vi "SetupFifo.vi"(8 "Force Num Array":i32, 9 "MaxNumFileWrite":i32=255, 10 "Fifo Time Out":i32=500, 11 "Fifo Size":u32=8192) -> (3 "Data Logging Param":T1)   [LabVIEW 2010, in "kevLib2010.lvlib"]
uses:
  kevLib2010.lvlib
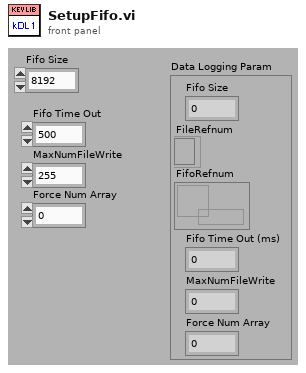
[diagram p1: front panel]
types:
  T1 = cluster{"Fifo Size":u32, "FileRefnum":refnum<file>, "FifoRefnum":refnum<k33>, "Fifo Time Out (ms)":i32, "MaxNumFileWrite":i32, "Force Num Array":i32}
  T2 = enum16{"open", "replace", "create", "open or create", "replace or create", "replace or create with confirmation"}
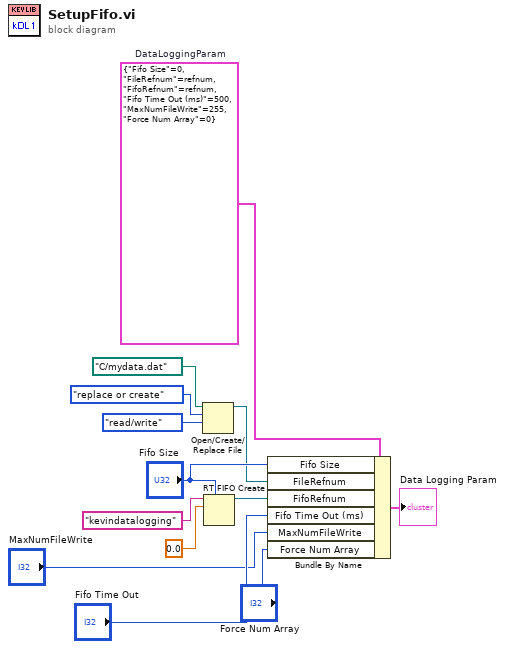
[diagram p0: block diagram]
diagram:
  w8 = T1 {"Fifo Size"=0, "FileRefnum"=refnum, "FifoRefnum"=refnum, "Fifo Time Out (ms)"=500, "MaxNumFileWrite"=255, "Force Num Array"=0}  # DataLoggingParam
  n1 = Open/Create/Replace File(file path (use dialog)=path "C:/mydata.dat", operation (0:open)=T2."replace or create", access (0:read/write)=enum16{"read/write", "read-only", "write-only"}."read/write") -> (refnum out=w6:refnum<file>)  [unwired: 3 in, 2 out]
  n2 = RT FIFO Create(0:"kevindatalogging" ("name (unnamed)"), 1:0.0, 4:"Fifo Size") -> (8:w5:refnum<k33>)  [unwired: 5 in, 2 out]
  n3 = Bundle By Name(cluster=w8, "Fifo Size"="Fifo Size", "FileRefnum"=w6, "FifoRefnum"=w5, "Fifo Time Out (ms)"="Fifo Time Out", "MaxNumFileWrite"="MaxNumFileWrite", "Force Num Array"="Force Num Array") -> (→"Data Logging Param":T1)
